vi "ArParser.vi"(1 "from\nXMLparser":string[][](array[string]), 2 "IndicatorClasses":string[](array[string]), 3 "IndicatorTypes":string[](array[string]), 4 "IndicatorNames":string[](array[string])) -> (0 "toCreator":T1(array[cluster]))   [LabVIEW 2017]
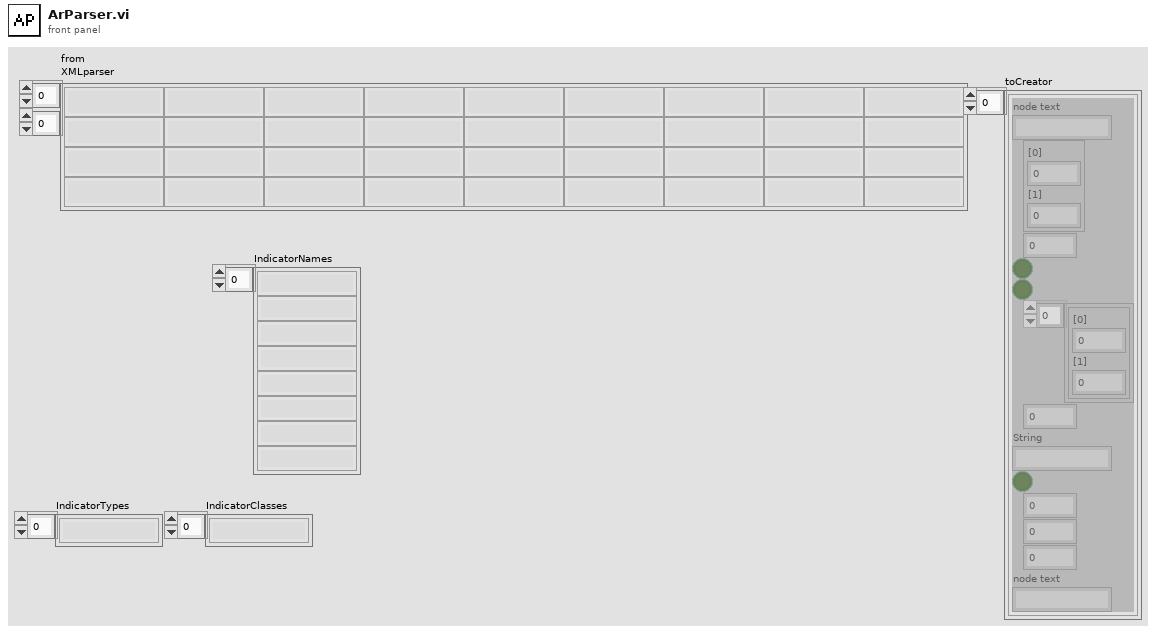
[diagram p1: front panel]
types:
  T1 = cluster{"node text":string, cluster{"[0]":i32, "[1]":i32}, i32, bool, bool, cluster{"[0]":u32, "[1]":u32}[], i32, "String":string, bool, i32, i32, i32, "node text":string}[]
  T2 = cluster{"node text":string, cluster{"[0]":i32, "[1]":i32}, i32, bool, bool, cluster{"[0]":u32, "[1]":u32}[], i32, "String":string, bool, i32, i32, i32, "node text":string}
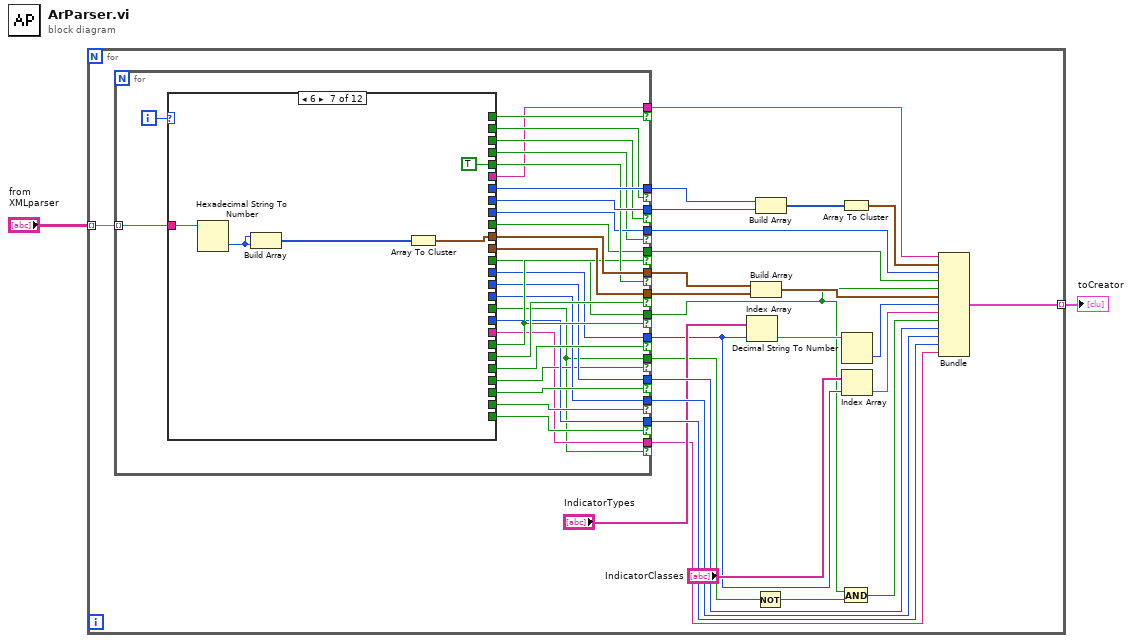
[diagram p0: block diagram]
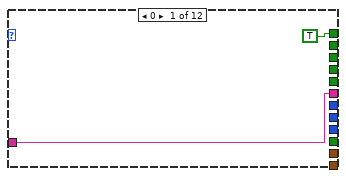
[diagram p2: hidden frame]
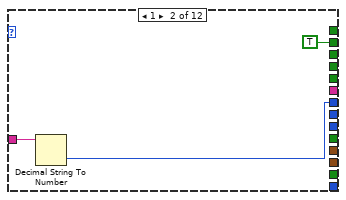
[diagram p3: hidden frame]
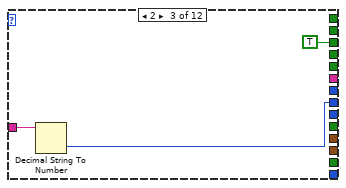
[diagram p4: hidden frame]
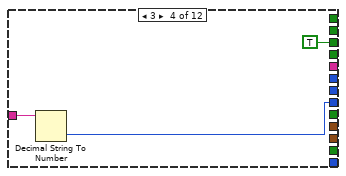
[diagram p5: hidden frame]
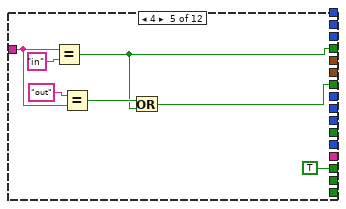
[diagram p6: hidden frame]
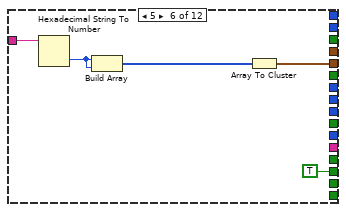
[diagram p7: hidden frame]
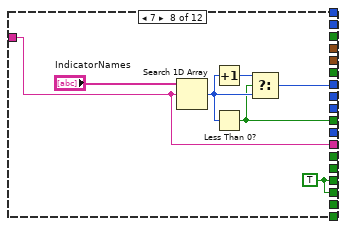
[diagram p8: hidden frame]
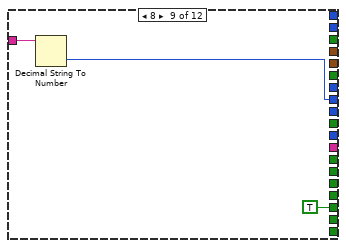
[diagram p9: hidden frame]
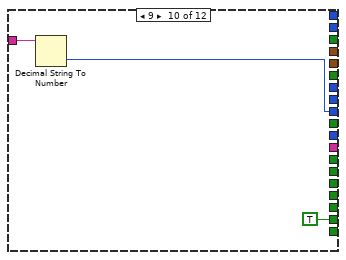
[diagram p10: hidden frame]
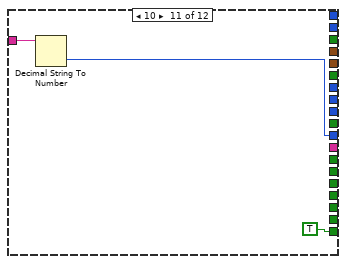
[diagram p11: hidden frame]
diagram:
  n1 = for {
    tunnel: "from\nXMLparser" -> [w28] mode=indexing
    tunnel: [w5] -> w1 mode=indexing
    n2 = for {
      tunnel: w28 -> [w56] mode=indexing
      tunnel: [w37] -> w4 if=w50
      tunnel: [w55] -> w18 if=w47
      tunnel: [w54] -> w17 if=w46
      tunnel: [w43] -> w27 if=w42
      tunnel: [w44] -> w26 if=w45
      tunnel: [w53] -> w21 if=w49
      tunnel: [w52] -> w20 if=w48
      tunnel: [w36] -> w7 if=w45
      tunnel: [w40] -> w12 if=w41
      tunnel: [w39] -> w25 if=w38
      tunnel: [w35] -> w24 if=w34
      tunnel: [w33] -> w23 if=w32
      tunnel: [w29] -> w9 if=w31
      tunnel: [w30] -> w3 if=w29
      i -> [w51]
      n3 = case shown="6" w51 {
        tunnel: w56 -> [w57 w61 w64 w67 w69 w79 w84 w88 w94 w97 w100 _]
        tunnel: [w57 _ _ _ _ _ _ _ _ _ _ _] -> w37
        tunnel: [_ w60 _ _ _ _ _ _ _ _ _ _] -> w55
        tunnel: [_ _ w63 _ _ _ _ _ _ _ _ _] -> w54
        tunnel: [_ _ _ w66 _ _ _ _ _ _ _ _] -> w43
        tunnel: [_ _ _ _ w68 _ _ _ _ _ _ _] -> w44
        tunnel: [_ _ _ _ _ w76 _ _ _ _ _ _] -> w53
        tunnel: [_ _ _ _ _ _ w81 _ _ _ _ _] -> w52
        tunnel: [TRUE _ _ _ _ _ _ _ _ _ _ _] -> w50
        tunnel: [_ _ _ _ TRUE _ _ _ _ _ _ _] -> w45
        tunnel: [_ _ _ _ _ TRUE _ _ _ _ _ _] -> w49
        tunnel: [_ _ _ _ _ _ TRUE _ _ _ _ _] -> w48
        tunnel: [_ TRUE _ _ _ _ _ _ _ _ _ _] -> w47
        tunnel: [_ _ TRUE _ _ _ _ _ _ _ _ _] -> w46
        tunnel: [_ _ _ TRUE _ _ _ _ _ _ _ _] -> w42
        tunnel: [_ _ _ _ w73 _ _ _ _ _ _ _] -> w36
        tunnel: [_ _ _ _ _ _ _ w90 _ _ _ _] -> w40
        tunnel: [_ _ _ _ _ _ _ w89 _ _ _ _] -> w41
        tunnel: [_ _ _ _ _ _ _ _ w93 _ _ _] -> w39
        tunnel: [_ _ _ _ _ _ _ _ TRUE _ _ _] -> w38
        tunnel: [_ _ _ _ _ _ _ _ _ w96 _ _] -> w35
        tunnel: [_ _ _ _ _ _ _ _ _ TRUE _ _] -> w34
        tunnel: [_ _ _ _ _ _ _ _ _ _ w99 _] -> w33
        tunnel: [_ _ _ _ _ _ _ _ _ _ TRUE _] -> w32
        tunnel: [_ _ _ _ _ _ _ w85 _ _ _ _] -> w29
        tunnel: [_ _ _ _ _ _ _ w89 _ _ _ _] -> w31
        tunnel: [_ _ _ _ _ _ _ w88 _ _ _ _] -> w30
        frame 0 {
        }
        frame 1 {
          n4 = Decimal String To Number(string=w61) -> (number=w60:i32)  [unwired: 2 in, 1 out]
        }
        frame 2 {
          n5 = Decimal String To Number(string=w64) -> (number=w63:i32)  [unwired: 2 in, 1 out]
        }
        frame 3 {
          n6 = Decimal String To Number(string=w67) -> (number=w66:i32)  [unwired: 2 in, 1 out]
        }
        frame 4 {
          n7 = Equal?(x=w69, y="in") -> (x = y?=w68:bool)
          n8 = Equal?(x="out", y=w69) -> (x = y?=w70:bool)
          n9 = Or(x=w70, y=w68) -> (x .or. y?=w73:bool)
        }
        frame 5 {
          n10 = Hexadecimal String To Number(string=w79) -> (number=w75:u32)  [unwired: 2 in, 1 out]
          n11 = Build Array(w75, w75) -> (w77:u32[])
          n12 = Array To Cluster(array=w77) -> (cluster=w76:cluster{"[0]":u32, "[1]":u32})
        }
        frame 6 {
          n13 = Hexadecimal String To Number(string=w84) -> (number=w80:u32)  [unwired: 2 in, 1 out]
          n14 = Build Array(w80, w80) -> (w82:u32[])
          n15 = Array To Cluster(array=w82) -> (cluster=w81:cluster{"[0]":u32, "[1]":u32})
        }
        frame 7 {
          w89 = TRUE
          n16 = Search 1D Array(1D array="IndicatorNames", element=w88) -> (index of element=w87:i32)  [unwired: 1 in]
          n17 = Increment(x=w87) -> (x+1=w86:i32)
          n18 = Less Than 0?(x=w87) -> (x < 0?=w85:bool)
          n19 = Select(t=w86, s=w85, f=w87) -> (s? t:f=w90:i32)
        }
        frame 8 {
          n20 = Decimal String To Number(string=w94) -> (number=w93:i32)  [unwired: 2 in, 1 out]
        }
        frame 9 {
          n21 = Decimal String To Number(string=w97) -> (number=w96:i32)  [unwired: 2 in, 1 out]
        }
        frame 10 {
          n22 = Decimal String To Number(string=w100) -> (number=w99:i32)  [unwired: 2 in, 1 out]
        }
        frame -1, Default {
        }
      }
    }
    n23 = Index Array(array="IndicatorTypes", index=w12) -> (element=w13:string)
    n24 = Build Array(w20, w21) -> (w22:cluster{"[0]":u32, "[1]":u32}[])
    n25 = Not(x=w9) -> (.not. x?=w8:bool)
    n26 = Build Array(w18, w17) -> (w19:i32[])
    n27 = Array To Cluster(array=w19) -> (cluster=w16:cluster{"[0]":i32, "[1]":i32})
    n28 = And(x=w7, y=w8) -> (x .and. y?=w6:bool)
    n29 = Decimal String To Number(string=w13) -> (number=w11:i32)  [unwired: 2 in, 1 out]
    n30 = Index Array(array="IndicatorClasses", index=w12) -> (element=w10:string)
    n31 = Bundle("node text"=w4, w16, w27, w26, w7, w22, w11, "String"=w10, w6, w25, w24, w23, "node text"=w3) -> (w5:T2)  [unwired: 1 in]
  }
  "toCreator" <- w1
